vi "Local gradient preallocation.vi"(9 "Image size":u32[](array[numeric]), 11 "R":dbl) -> (1 "Sizes":T2, 3 "FFT":T1)   [LabVIEW 2015]
doc: "Calculates preallocations for local gradient. Takes window size (R) and Image size as an input. Outputs FFT of X, Y gradient and SUM kernels.\n\nAlso provides sizes used for FFT calculations which are required to correctly calculate the inverse Fourier transform\n\nAuthor: Anatolii Kashchuk"
uses:
  <vilib>/Analysis/2dsp.llb/2D Real FFT.vi
  <vilib>/Analysis/NI_AALPro.lvlib
panel:
  # "Author: Anatolii Kashchuk"
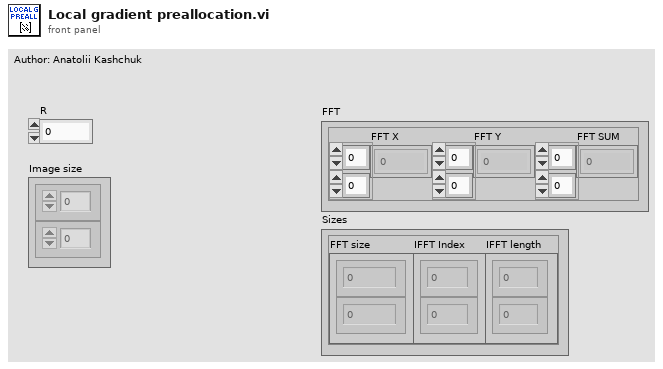
[diagram p1: front panel]
types:
  T1 = cluster{"FFT SUM":cdb[][], "FFT X":cdb[][], "FFT Y":cdb[][]}
  T2 = cluster{"FFT size":u32[], "IFFT Index":i32[], "IFFT length":u32[]}
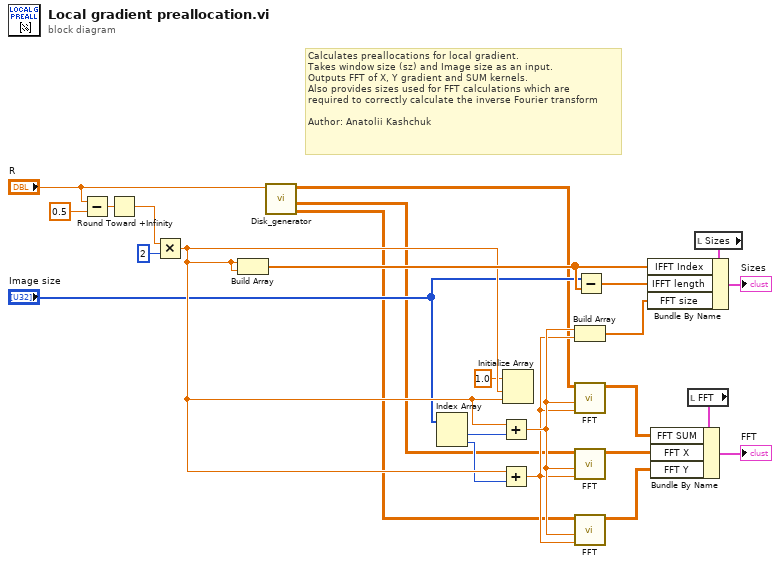
[diagram p0: block diagram]
diagram:
  # "Calculates preallocations for local gradient.\nTakes window size (sz) and Image size as an input.\nOutputs FFT of X, Y gradient and SUM kernels.\nAlso provides sizes used for FFT calculations which are \nrequired to correctly calculate the inverse Fourier transform\n\nAuthor: Anatolii Kashchuk"
  n1 = Subtract(x="R", y=0.5) -> (x-y=w2:dbl)
  n2 = Round Toward +Infinity(x=w2) -> (ceil(x): smallest int >= x=w1:dbl)
  n3 = Multiply(x=w1, y=u32 2) -> (x*y=w24:dbl)
  n4 = Build Array(w24, w24) -> (w25:dbl[])
  n5 = call "Disk_generator.vi"("r"="R") -> ("GradY"=w8:dbl[][], "GradX"=w5:dbl[][], "disk"=w6:dbl[][])  [unwired: 8 in]
  n6 = Index Array(array="Image size") -> (element #1=w21:u32, element #2=w22:u32)  [unwired: 2 in]
  n7 = Add(x=w24, y=w21) -> (x+y=w17:dbl)
  n8 = Add(x=w24, y=w22) -> (x+y=w16:dbl)
  n9 = Initialize Array(1.0 ("element"), w24, w24) -> ()  [unwired: 1 out]
  n10 = Build Array(w17, w16) -> (w15:dbl[])
  n11 = call-poly <vilib>:"FFT.vi"("n"=w16, "m"=w17, "X"=w6) -> ("FFT {X}"=w7:cdb[][])  [unwired: 7 in, 1 out]
  n12 = call-poly <vilib>:"FFT.vi"("n"=w16, "m"=w17, "X"=w5) -> ("FFT {X}"=w14:cdb[][])  [unwired: 7 in, 1 out]
  n13 = call-poly <vilib>:"FFT.vi"("n"=w16, "m"=w17, "X"=w8) -> ("FFT {X}"=w13:cdb[][])  [unwired: 7 in, 1 out]
  n14 = Subtract(x="Image size", y=w25) -> (x-y=w23:dbl[])
  n15 = local read "FFT"() -> (w10:T1)
  n16 = Bundle By Name(cluster=w10, "FFT SUM"=w7, "FFT X"=w14, "FFT Y"=w13) -> (→"FFT":T1)
  n17 = local read "Sizes"() -> (w12:T2)
  n18 = Bundle By Name(cluster=w12, "IFFT Index"=w25, "IFFT length"=w23, "FFT size"=w15) -> (→"Sizes":T2)
